vi "Get Digital Value.vi"(7 "GPIO":i32, 8 "error in (no error)":errorcluster, 11 "VISA resource name in":refnum<visa-resource-name>) -> (0 "error out":errorcluster, 1 "Value":bool, 3 "VISA resource name":refnum<visa-resource-name>)   [LabVIEW 2024, in "CTIPicoVISA.lvlib"]
uses:
  CTIPicoVISA.lvlib
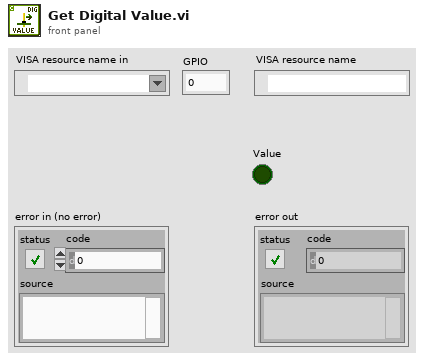
[diagram p1: front panel]
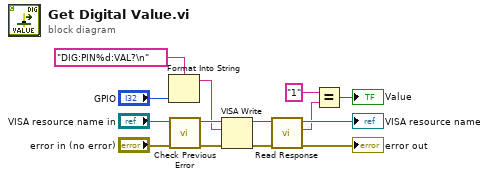
[diagram p0: block diagram]
diagram:
  n1 = Format Into String(format string="DIG:PIN%d:VAL?\n", "GPIO") -> (resulting string=w9:string)  [unwired: 2 in, 1 out]
  n2 = call "Check Previous Error.vi"("error in (no error)"="error in (no error)", "VISA resource name in"="VISA resource name in") -> ("error out"=w10:errorcluster, "VISA resource name"=w11:refnum<visa-resource-name>)  [unwired: 8 in]
  n3 = VISA Write(VISA resource name=w11, write buffer=w9, error in (no error)=w10) -> (VISA resource name out=w2:refnum<visa-resource-name>, error out=w8:errorcluster)  [unwired: 1 out]
  n4 = call "Read Response.vi"("error in (no error)"=w8, "VISA resource name"=w2) -> ("error out"=→"error out":errorcluster, "Response"=w5:string, "VISA resource name Out"=→"VISA resource name":refnum<visa-resource-name>)  [unwired: 6 in, 1 out]
  n5 = Equal?(x="1", y=w5) -> (x = y?=→"Value":bool)
